vi "Streamline.vi"(4 "Properties":T1={"Density"=nan, "Arrow Size"=nan, "Line"={"Style"=enum."Automatic", "Color"=2147483647, "Width"=nan}, "Colormap"={"Map"=enum."Automatic", "Value Min"=nan, "Value Max"=nan, "Scaling"=enum."Default", "Reverse"=FALSE}} {"Line"."Color" items=["Automatic"=2147483647, "Black"=0, "White"=16777215, "Red"=16711680, "Green"=2263842, "Blue"=255, "Cyan"=65535, "Magenta"=16711935, "Yellow"=16776960]}, 5 "Y Vector Component":dbl[][](array[numeric]), 6 "Colormap Value":dbl[][](array[numeric]), 7 "X Vector Component":dbl[][](array[numeric]), 8 "error in (no error)":errorcluster, 9 "Y Coordinates":dbl[](array[numeric]), 10 "X Coordinates":dbl[](array[numeric]), 11 "Plot ID":T8 format="%x") -> (0 "error out":errorcluster, 3 "Plot ID Out":T8 format="%x")   [LabVIEW 2013, in "Advanced Plotting Toolkit.lvlib"]
doc: "Display a vector field using streamlines. Provide two 2D arrays, one giving the X component of the vector field at each point, and the other giving the Y component."
uses:
  Advanced Plotting Toolkit.lvlib
  typedefs/PlotID.ctl
  StreamlineProperties.ctl
  properties/Line.ctl
  properties/Line_Style.ctl
  typedefs/PlotColor.ctl
  properties/Colormap.ctl
  properties/Colormap_Map.ctl
  properties/Colormap_Scaling.ctl
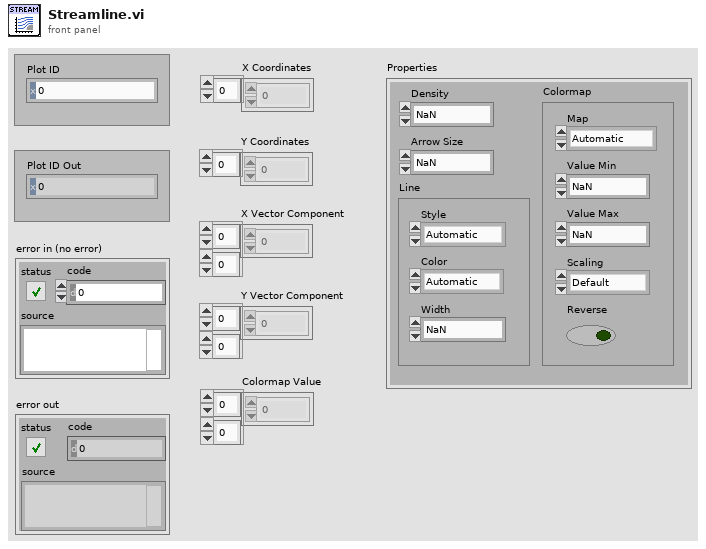
[diagram p1: front panel]
types:
  T1 = typedef "Advanced Plotting Toolkit.lvlib/StreamlineProperties.ctl" = cluster{"Density":dbl, "Arrow Size":dbl, "Line":T2, "Colormap":T5}
  T2 = typedef "Advanced Plotting Toolkit.lvlib/Line.ctl" = cluster{"Style":T3, "Color":T4, "Width":sgl}
  T3 = typedef "Advanced Plotting Toolkit.lvlib/Line_Style.ctl" = enum16{"Automatic", "Solid", "Dashed", "Dotted", "Dash-dot", "Invisible"}
  T4 = typedef "Advanced Plotting Toolkit.lvlib/PlotColor.ctl" = u32
  T5 = typedef "Advanced Plotting Toolkit.lvlib/Colormap.ctl" = cluster{"Map":T6, "Value Min":dbl, "Value Max":dbl, "Scaling":T7, "Reverse":bool}
  T6 = typedef "Advanced Plotting Toolkit.lvlib/Colormap_Map.ctl" = enum16{"Automatic", "Rainbow", "Hot and Cold", "White-Black", "White-Blue", "White-Green", "White-Red", "Fire", "Water", "Earth", "Air", "Pastel", "Banded", "Stepped"}
  T7 = typedef "Advanced Plotting Toolkit.lvlib/Colormap_Scaling.ctl" = enum16{"Default"}
  T8 = typedef "Advanced Plotting Toolkit.lvlib/PlotID.ctl" = i32
  T9 = typedef "Advanced Plotting Toolkit.lvlib/KeyValue.ctl" = cluster{"Key":string, "Value":string}
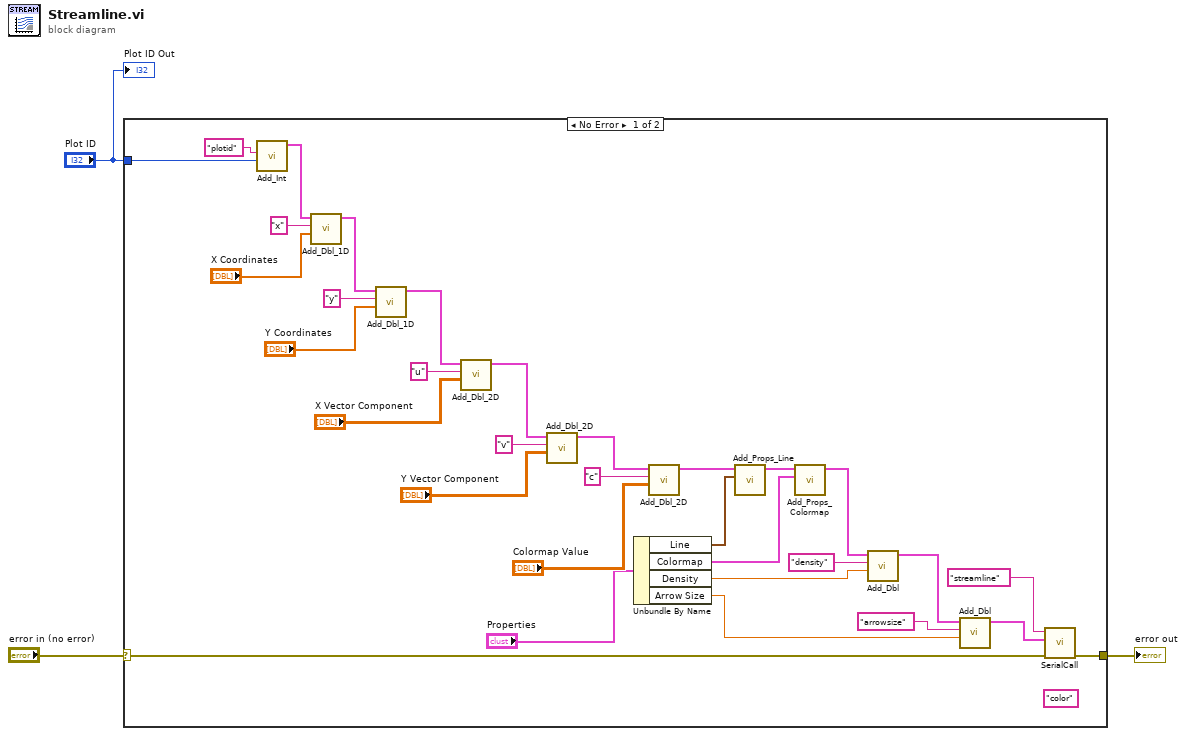
[diagram p0: block diagram]
diagram:
  n1 = case shown="No Error" "error in (no error)" {
    selector: "error in (no error)" -> [w16 w36]
    tunnel: "Plot ID" -> [w35 _]
    tunnel: [w15 w36] -> w1
    frame No Error {
      (unwired) "color" ("Key")
      n2 = call "Add_Int.vi"("Value"=w35, "Key"="plotid") -> ("Keyword Array Out"=w33:T9[])  [unwired: 9 in]
      n3 = call "Add_Dbl_1D.vi"("Value"="X Coordinates", "Key"="x", "Keyword Array"=w33) -> ("Keyword Array Out"=w29:T9[])  [unwired: 8 in]
      n4 = call "Add_Dbl_1D.vi"("Value"="Y Coordinates", "Key"="y", "Keyword Array"=w29) -> ("Keyword Array Out"=w27:T9[])  [unwired: 8 in]
      n5 = call "Add_Dbl_2D.vi"("Value"="X Vector Component", "Key"="u", "Keyword Array"=w27) -> ("Keyword Array Out"=w23:T9[])  [unwired: 8 in]
      n6 = call "Add_Dbl_2D.vi"("Value"="Y Vector Component", "Key"="v", "Keyword Array"=w23) -> ("Keyword Array Out"=w21:T9[])  [unwired: 8 in]
      n7 = Unbundle By Name("Properties") -> ("Line"=w11:T2, "Colormap"=w14:T5, "Density"=w10:dbl, "Arrow Size"=w7:dbl)
      n8 = call "Add_Dbl_2D.vi"("Value"="Colormap Value", "Key"="c", "Keyword Array"=w21) -> ("Keyword Array Out"=w13:T9[])  [unwired: 8 in]
      n9 = call "Add_Props_Line.vi"("Line"=w11, "Keyword Array"=w13) -> ("Keyword Array Out"=w12:T9[])  [unwired: 9 in]
      n10 = call "Add_Props_Colormap.vi"("Colormap"=w14, "Keyword Array"=w12) -> ("Keyword Array Out"=w6:T9[])  [unwired: 9 in]
      n11 = call "Add_Dbl.vi"("Value"=w10, "Key"="density", "Keyword Array"=w6) -> ("Keyword Array Out"=w5:T9[])  [unwired: 8 in]
      n12 = call "Add_Dbl.vi"("Value"=w7, "Key"="arrowsize", "Keyword Array"=w5) -> ("Keyword Array Out"=w4:T9[])  [unwired: 8 in]
      n13 = call "SerialCall.vi"("error in (no error)"=w16, "data"=w4, "Resource"="streamline") -> ("error out"=w15:errorcluster)  [unwired: 7 in, 1 out]
    }
    frame Error {
    }
  }
  "error out" <- w1
  "Plot ID Out" <- "Plot ID"
